vi "final_usrp_transceiver.vi"() -> ()   [LabVIEW 2014]
uses:
  <vilib>/vision/Image Controls.llb/IMAQ Image.ctl
  <vilib>/addons/Modulation/Analog/support/mod_Set Error Source.vi
  var_stop.vi
  <vilib>/addons/Modulation/Digital/Support/Common/Validators/mod_Generate Filter Coefficients Validate.vi
  <vilib>/addons/Modulation/Digital/General/subVIs/mod_Generate Filter Coefficients.vi
  <vilib>/measure/maspectr.llb/FFT Power Spectrum and PSD for 1 Chan (CDB).vi
  <vilib>/addons/Modulation/Digital/General/MT Apply Matched Filter (Generic).vi
  <vilib>/addons/Modulation/Digital/General/MT Align to Ideal Symbols (Generic).vi
  <instrlib>/niUSRP/niUSRP Fetch Rx Data (CDB Cluster).vi
  <instrlib>/niUSRP/niUSRP Write Tx Data (CDB Cluster).vi
  <vilib>/addons/Modulation/Digital/General/MT Apply Pulse Shaping Filter (Generic).vi
  <vilib>/addons/Modulation/niDMT.lvlib
  <vilib>/measure/NI_MAPro.lvlib
panel:
  out "size(s) 4":i32
  out "length 2":i32
  out "frame num":u32
  out "length":i32[](array[numeric])
  out "start index":i32[](array[numeric])
  out "Numeric":i32
  out "size(s) 3":i32
  out "# elements in queue 2":i32
  out "size(s) 2":i32
  out "size(s)":i32[](array[numeric])
  out "image":T1(plugin-control)
  in  "Transmit power (db)":dbl
  out "found?":bool
  out "# elements in queue":i32
  out "Spectrum monitor":cluster{"f0":dbl, "df":dbl, "magnitude":dbl[]}(graph)={"f0"=-0.49993781867926873, "df"=0.00012436264146250465, "magnitude"=[]}
  out "RX Constellation Map":cdb[](graph)
  out "valid?":bool
  in  "Gray code?":bool
  in  "Modulation":enum16{"PSK", "QAM"}(ring)=enum."QAM"
  out "packet len":u32
  in  "filter length (symbols)":i32=8
  in  "filter parameter":dbl=0.5 format="%.2f"
  in  "pulse shaping filter (none)":T2(ring)=enum."Raised Cosine"
  in  "M-PSK (4)":i32=16 caption="M-ARY"
  in  "samples per symbol (16)":i32=4
  out "packet bits length":i32
  in  "number of samples":i64=40000
  out "RX coerced gain":dbl format="%#_6f"
  out "RX coerced carrier frequency":dbl=915000000.0 format="%#_6p"
  out "RX coerced IQ rate":dbl=4000000.0 format="%#_6p"
  in  "RX active antenna":string="RX2"
  in  "RX gain":dbl format="%#_6f"
  in  "RX device names":refnum<k15>="192.168.10.2"
  out "TX coerced gain":dbl format="%#_6f"
  out "TX coerced carrier frequency":dbl=915000000.0 format="%#_6p"
  out "coerced IQ rate":dbl=4000000.0 format="%#_6p"
  in  "TX device names":refnum<k15>="192.168.10.2"
  in  "TX gain":dbl format="%#_6f"
  in  "carrier frequency":dbl=915000000.0 format="%#_6p"
  in  "IQ rate":dbl=800000.0 format="%#_6p"
  in  "stop":bool
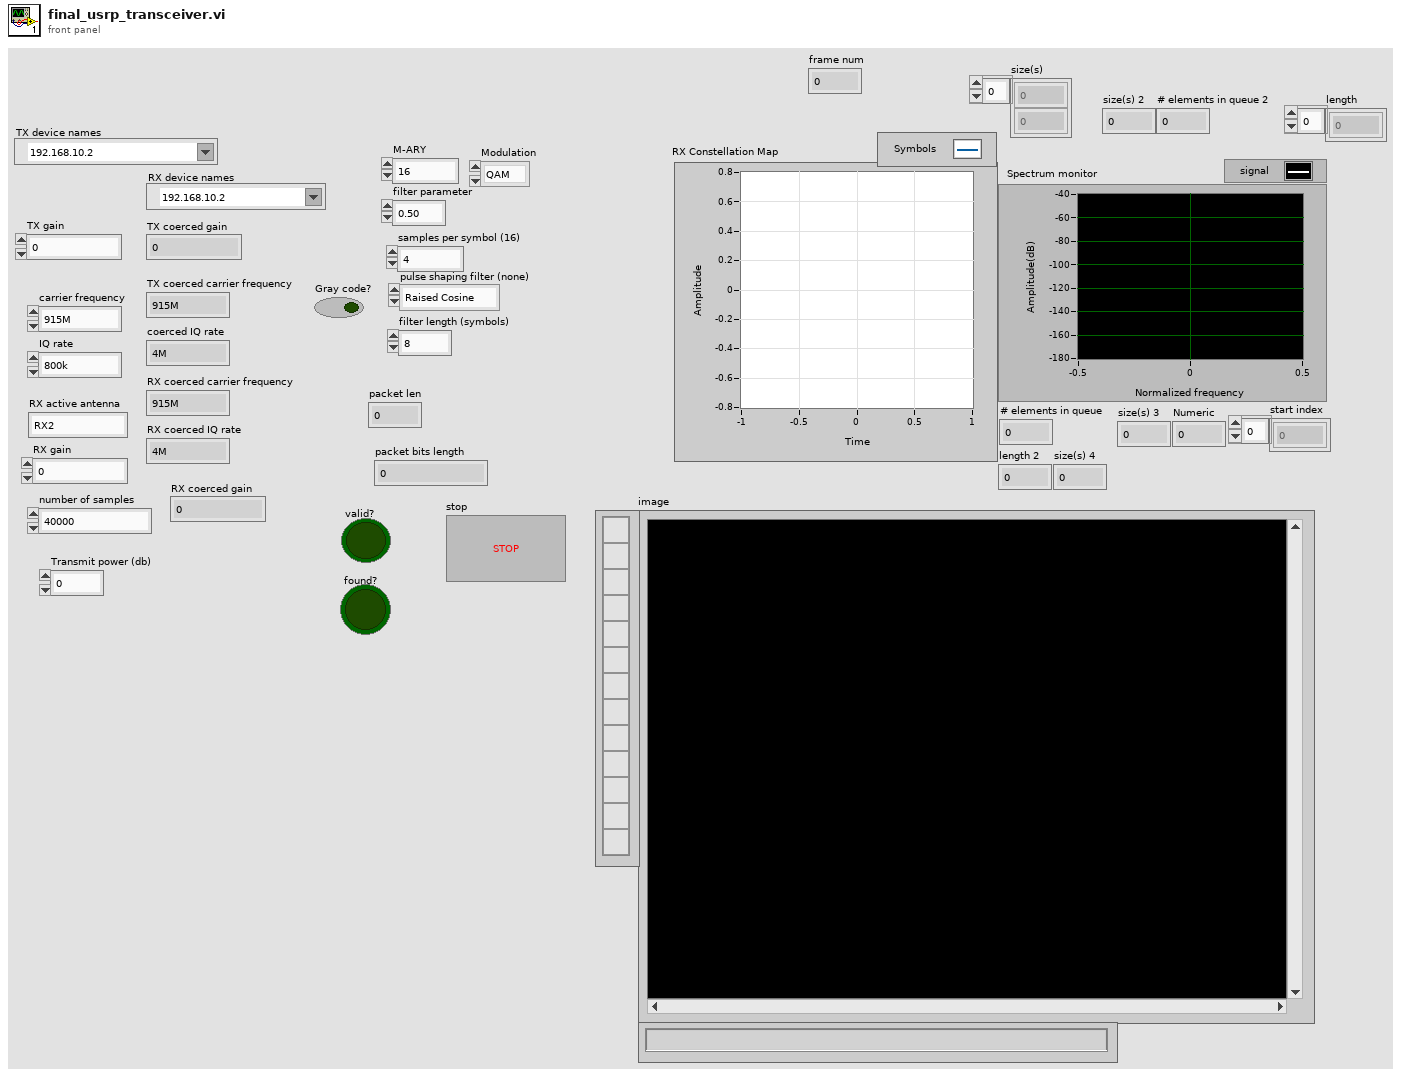
[diagram p1: front panel]
types:
  T1 = typedef "IMAQ Image.ctl" = refnum<image>
  T2 = enum16{"none", "Raised Cosine", "Root Raised Cos", "Gaussian"}
  T3 = enum16{"FSK", "PSK", "QAM", "MSK", "PAM", "ASK", "CPM"}
  T4 = cluster{"samples per symbol (16)":i32, "symbol map":cdb[], "index map":u32[]}
  T5 = cluster{"samples per symbol (16)":i32, "symbol map":cdb[], i32[]}
  T6 = typedef "niAMT.lvlib/Complex Data Waveform.ctl" = cluster{"t0":dbl, "dt":dbl, "Y":cdb[]}
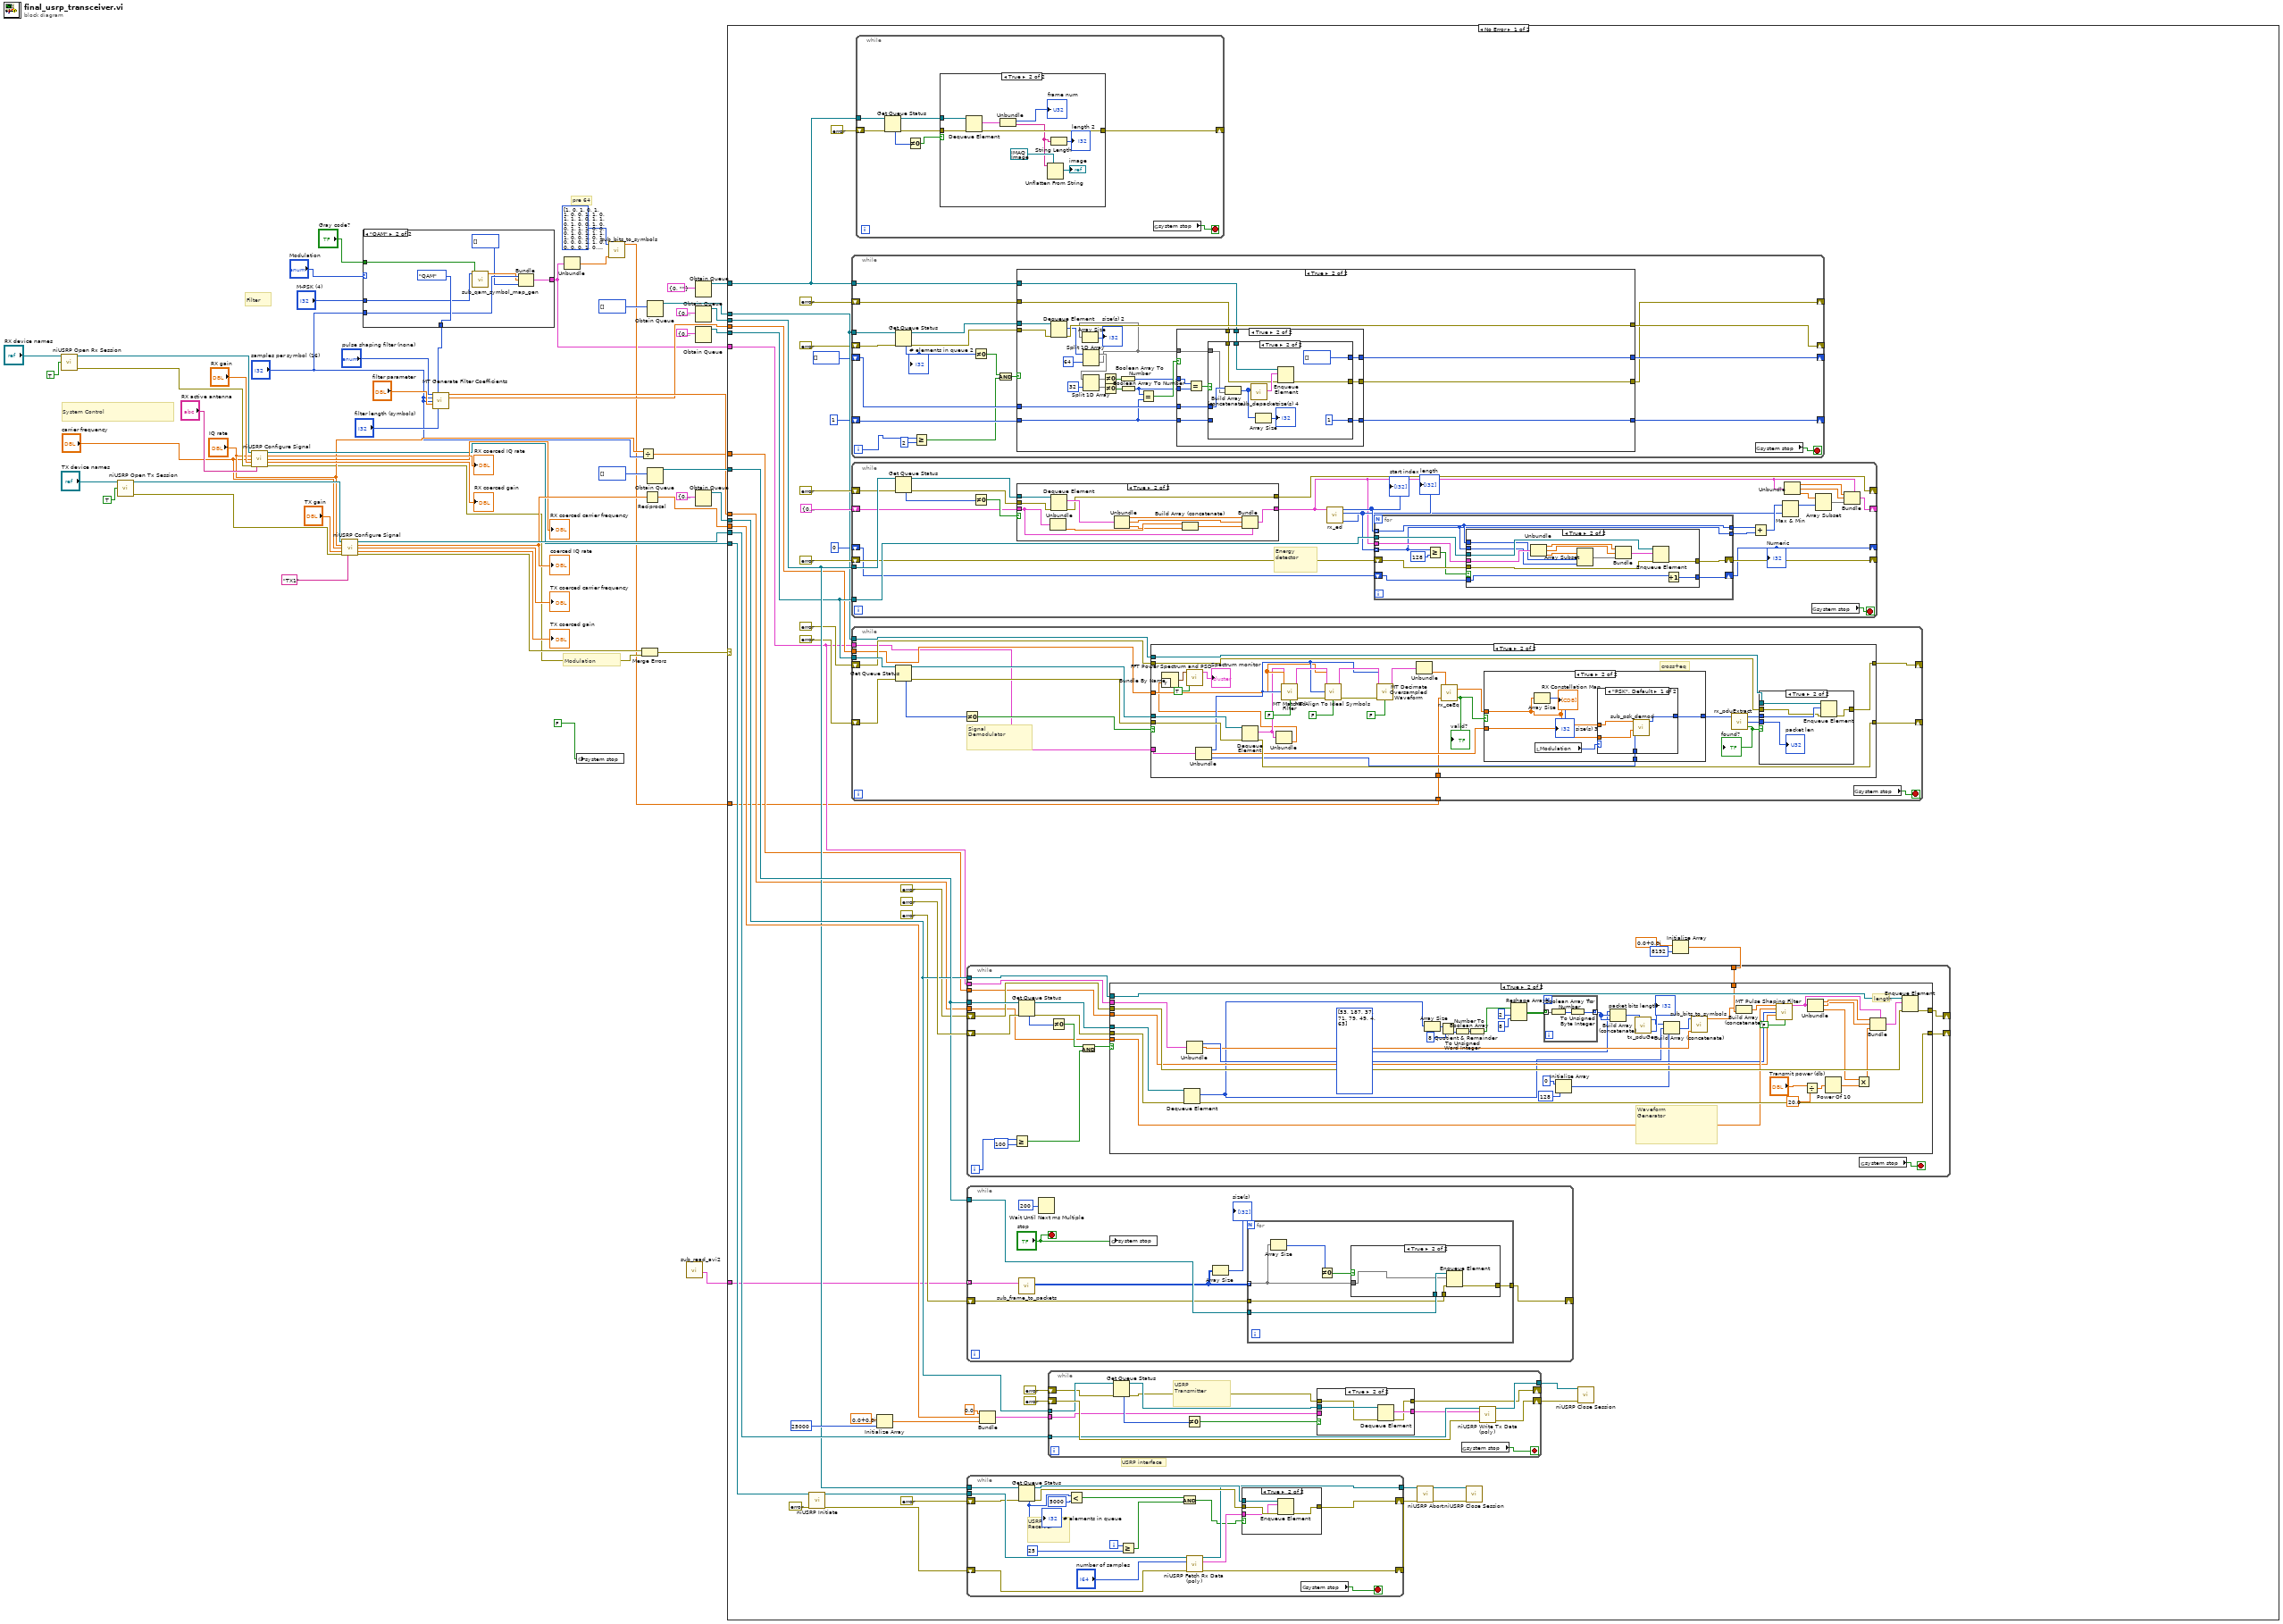
[diagram p0: block diagram]
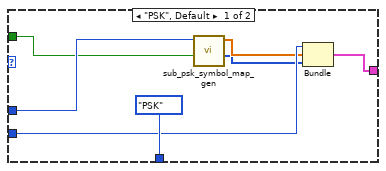
[diagram p2: hidden frame]
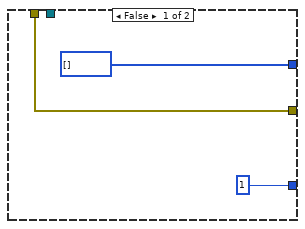
[diagram p5: hidden frame]
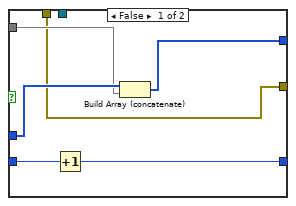
[diagram p6: hidden frame]
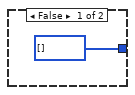
[diagram p8: hidden frame]
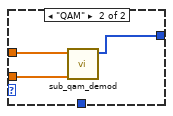
[diagram p9: hidden frame]
diagram:
  # "pre 64"
  # "Modulation"
  # "Filter"
  # "System Control"
  n1 = call <instrlib>:"niUSRP Open Rx Session.vi"("device names"="RX device names", "reset"=TRUE) -> ("session handle out"=w41:refnum<k15>, "error out"=w40:errorcluster)  [unwired: 12 in]
  n2 = call <instrlib>:"niUSRP Open Tx Session.vi"("device names"="TX device names", "reset"=TRUE) -> ("session handle out"=w54:refnum<k15>, "error out"=w53:errorcluster)  [unwired: 12 in]
  n3 = call <instrlib>:"niUSRP Configure Signal.vi"("session handle"=w41, "IQ rate"="IQ rate", "carrier frequency"="carrier frequency", "gain"="RX gain", "error in (no error)"=w40, "active antenna"="RX active antenna") -> ("session handle out"=w32:refnum<k15>, "coerced IQ rate"=→"RX coerced IQ rate":dbl, "coerced carrier frequency"=→"RX coerced carrier frequency":dbl, "coerced gain"=→"RX coerced gain":dbl, "error out"=w16:errorcluster)  [unwired: 5 in]
  n4 = call <instrlib>:"niUSRP Configure Signal.vi"("session handle"=w54, "IQ rate"="IQ rate", "carrier frequency"="carrier frequency", "gain"="TX gain", "error in (no error)"=w53, "active antenna"="TX1") -> ("session handle out"=w45:refnum<k15>, "coerced IQ rate"=w43:dbl, "coerced carrier frequency"=→"TX coerced carrier frequency":dbl, "coerced gain"=→"TX coerced gain":dbl, "error out"=w17:errorcluster)  [unwired: 5 in]
  "coerced IQ rate" <- w43
  n5 = case shown="\"QAM\"" "Modulation" {
    tunnel: [T3."PSK" ("modulation type") T3."QAM" ("modulation type")] -> w11
    tunnel: "M-PSK (4)" -> [w61 w67]
    tunnel: "Gray code?" -> [w60 w68]
    tunnel: "samples per symbol (16)" -> [w59 w66]
    tunnel: [w56 w63] -> w4
    frame "PSK", Default {
      n6 = call "sub_psk_symbol_map_gen.vi"("Gray code?"=w60, "M-PSK"=w61) -> ("index map"=w57:u32[], "symbol map"=w58:cdb[])  [unwired: 8 in]
      n7 = Bundle("samples per symbol (16)"=w59, "symbol map"=w58, "index map"=w57) -> (w56:T4)  [unwired: 1 in]
    }
    frame "QAM" {
      n8 = call "sub_qam_symbol_map_gen.vi"("Gray code?"=w68, "M-QAM"=w67) -> ("symbol map"=w65:cdb[])  [unwired: 9 in]
      n9 = Bundle("samples per symbol (16)"=w66, "symbol map"=w65, i32[] []) -> (w63:T5)  [unwired: 1 in]
    }
  }
  n10 = call <vilib>:"MT Generate Filter Coefficients.vi"("pulse shaping filter (none)"="pulse shaping filter (none)", "modulation type"=w11, "pulse shaping samples per symbol (16)"="samples per symbol (16)", "matched samples per symbol (16)"="samples per symbol (16)", "filter parameter"="filter parameter", "filter length (symbols)"="filter length (symbols)") -> ("pulse shaping filter coefficients"=w22:dbl[], "matched filter coefficients"=w20:dbl[])  [unwired: 7 in, 1 out]
  n11 = Unbundle(w4) -> ("symbol map"=w6:cdb[])  [unwired: 2 out]
  n12 = global write "var_stop.vi" "system stop"(FALSE) -> ()
  n13 = call "sub_bits_to_symbols.vi"("symbol map"=w6, "bits"=i16[] [1, 0, 1, 0, 1, 1, 0, 0, 1, 1, 0, 1, 1, 1, 0, 1, 1, 0, 1, 0, 0, 1, 0, 0, 1, 1, 1, 0, 0, 0, 1, 0, 1, 1, 1, 1, 0, 0, 1, 0, 1, 0, 0, 0, 1, 1, 0, 0, 0, 0, 1, 0, 0, 0, 0, 0, 1, 1, 1, 1, 1, 1, 0, 0] ("preamble(64) 2")) -> ("symbols"=w5:cdb[])  [unwired: 9 in]
  n14 = Divide(x="IQ rate", y="samples per symbol (16)") -> (x/y=w21:dbl)
  n15 = Merge Errors(w17, w16) -> (w15:errorcluster)
  n16 = Reciprocal(x=w43) -> (1/x=w42:dbl)
  n17 = Obtain Queue(element data type=i8[] [] ("output bit stream")) -> (queue out=w27:refnum<queue>)  [unwired: 4 in, 2 out]
  n18 = Obtain Queue(element data type=i16[] []) -> (queue out=w55:refnum<queue>)  [unwired: 4 in, 2 out]
  n19 = call "sub_read_avi2.vi"() -> ("frames"=w3:cluster{i32, "Data String":string}[])  [unwired: 10 in, 1 out]
  n20 = Obtain Queue(element data type=cluster{u32, "string":string} {0, "string"=""} ("frame")) -> (queue out=w1:refnum<queue>)  [unwired: 4 in, 2 out]
  n21 = Obtain Queue(element data type=cluster{"t0":dbl, "dt":dbl, "Y":cdb[]} {"t0"=0.0, "dt"=0.0, "Y"=[]} ("data")) -> (queue out=w31:refnum<queue>)  [unwired: 4 in, 2 out]
  n22 = Obtain Queue(element data type=cluster{"t0":dbl, "dt":dbl, "Y":cdb[]} {"t0"=0.0, "dt"=0.0, "Y"=[]} ("data")) -> (queue out=w28:refnum<queue>)  [unwired: 4 in, 2 out]
  n23 = Obtain Queue(element data type=cluster{"t0":dbl, "dt":dbl, "Y":cdb[]} {"t0"=0.0, "dt"=1.0, "Y"=[]} ("data")) -> (queue out=w46:refnum<queue>)  [unwired: 4 in, 2 out]
  n24 = case shown="No Error" w15 {
    tunnel: w55 -> [w117 _]
    tunnel: w46 -> [w112 _]
    tunnel: w45 -> [w113 _]
    tunnel: w42 -> [w106 _]
    tunnel: w32 -> [w101 _]
    tunnel: w31 -> [w95 _]
    tunnel: w28 -> [w91 _]
    tunnel: w27 -> [w89 _]
    tunnel: w4 -> [w83 _]
    tunnel: w22 -> [w86 _]
    tunnel: w21 -> [w85 _]
    tunnel: w20 -> [w84 _]
    tunnel: w5 -> [w77 _]
    tunnel: w3 -> [w76 _]
    tunnel: w1 -> [w72 _]
    frame No Error {
      # "USRP interface"
      n25 = call <instrlib>:"niUSRP Initiate.vi"("session handle"=w101, "error in (no error)"=errorcluster {"status"=FALSE, "code"=0, "source"=""}) -> ("session handle out"=w100:refnum<k15>, "error out"=w99:errorcluster)  [unwired: 12 in]
      n26 = while {
        tunnel: w89 -> [w155]
        shift-right: [w148] -> _
        shift-left: errorcluster {"status"=FALSE, "code"=0, "source"=""} ("error out") -> [w154]
        shift-right: [w146] -> _
        shift-left: u32 1 -> [w147]
        shift-right: [w145] -> _
        shift-left: i8[] [] ("second subarray") -> [w144]
        tunnel: w72 -> [w143]
        shift-right: [w141] -> _
        shift-left: errorcluster {"status"=FALSE, "code"=0, "source"=""} ("error out") -> [w142]
        i -> [w139]
        stop <- w153 stop-if-true
        n27 = Get Queue Status(queue=w155, error in (no error)=w154) -> (queue out=w150:refnum<queue>, error out=w149:errorcluster, # elements in queue=w152:i32)  [unwired: 1 in, 5 out]
        "# elements in queue 2" <- w152
        n28 = Greater Or Equal?(x=w139, y=2) -> (x >= y?=w138:bool)
        n29 = Not Equal To 0?(x=w152) -> (x != 0?=w151:bool)
        n30 = And(x=w151, y=w138) -> (x .and. y?=w137:bool)
        n31 = case shown="True" w137 {
          tunnel: w150 -> [_ w182]
          tunnel: w149 -> [w159 w181]
          tunnel: [w159 w180] -> w148
          tunnel: w147 -> [w158 w166]
          tunnel: [w158 w167] -> w146
          tunnel: [w156 w171] -> w145
          tunnel: w144 -> [w156 w168]
          tunnel: w143 -> [_ w165]
          tunnel: w142 -> [w157 w164]
          tunnel: [w157 w163] -> w141
          frame False {
          }
          frame True {
            n32 = Dequeue Element(queue=w182, error in (no error)=w181) -> (element=w162:i8[], error out=w180:errorcluster)  [unwired: 1 in, 2 out]
            n33 = Split 1D Array(array=w162, index=64) -> (first subarray=w173:i8[], second subarray=w160:i8[])
            n34 = Array Size(array=w160) -> (size(s)=→"size(s) 2":i32)
            n35 = Split 1D Array(array=w173, index=32) -> (first subarray=w176:i8[], second subarray=w177:i8[])
            n36 = Not Equal To 0?(x=w176) -> (x != 0?=w175:bool[])
            n37 = Not Equal To 0?(x=w177) -> (x != 0?=w174:bool[])
            n38 = Boolean Array To Number(Boolean array=w175) -> (number=w170:u32)
            n39 = Boolean Array To Number(Boolean array=w174) -> (number=w169:u32)
            n40 = Equal?(x=w169, y=w166) -> (x = y?=w172:bool)
            n41 = case shown="True" w172 {
              tunnel: [i8[] [] ("second subarray") w193] -> w171
              tunnel: w170 -> [_ w196]
              tunnel: w169 -> [_ w195]
              tunnel: w168 -> [_ w192]
              tunnel: w160 -> [_ w191]
              tunnel: [u32 1 w190] -> w167
              tunnel: w166 -> [_ w189]
              tunnel: w165 -> [_ w188]
              tunnel: w164 -> [w183 w187]
              tunnel: [w183 w186] -> w163
              frame False {
              }
              frame True {
                n42 = Equal?(x=w196, y=w195) -> (x = y?=w194:bool)
                n43 = case shown="True" w194 {
                  tunnel: [w200 i8[] [] ("second subarray")] -> w193
                  tunnel: w192 -> [w202 w210]
                  tunnel: w191 -> [w201 w209]
                  tunnel: [w198 u32 1] -> w190
                  tunnel: w189 -> [w199 _]
                  tunnel: w188 -> [_ w208]
                  tunnel: w187 -> [w197 w206]
                  tunnel: [w197 w205] -> w186
                  frame False {
                    n44 = Increment(x=w199) -> (x+1=w198:u32)
                    n45 = Build Array (concatenate)(w202, w201) -> (w200:i8[])
                  }
                  frame True {
                    n46 = Build Array (concatenate)(w210, w209) -> (w204:i8[])
                    n47 = call "sub_depacket.vi"("bitstream"=w204) -> ("frame"=w207:cluster{u32, "string":string})  [unwired: 10 in]
                    n48 = Array Size(array=w204) -> (size(s)=→"size(s) 4":i32)
                    n49 = Enqueue Element(queue=w208, element=w207, error in (no error)=w206) -> (error out=w205:errorcluster)  [unwired: 1 in, 2 out]
                  }
                }
              }
            }
          }
        }
        n50 = global read "var_stop.vi" "system stop"() -> (w153:bool)
      }
      n51 = while {
        tunnel: w95 -> [w307]
        shift-right: [w300] -> _
        shift-left: errorcluster {"status"=FALSE, "code"=0, "source"=""} ("error out") -> [w306]
        shift-right: [w286] -> _
        shift-left: cluster{"t0":dbl, "dt":dbl, "Y":cdb[]} {"t0"=0.0, "dt"=0.0, "Y"=[]} ("data") -> [w301]
        tunnel: w91 -> [w299]
        shift-right: [w298] -> _
        shift-left: errorcluster {"status"=FALSE, "code"=0, "source"=""} ("error out") -> [w297]
        shift-right: [w281] -> _
        shift-left: 0 -> [w282]
        stop <- w296 stop-if-true
        # "Energy\ndetector"
        n52 = Get Queue Status(queue=w307, error in (no error)=w306) -> (queue out=w302:refnum<queue>, error out=w303:errorcluster, # elements in queue=w305:i32)  [unwired: 1 in, 5 out]
        n53 = Not Equal To 0?(x=w305) -> (x != 0?=w304:bool)
        n54 = case shown="True" w304 {
          tunnel: w303 -> [w334 w345]
          tunnel: w302 -> [_ w344]
          tunnel: w301 -> [w333 w339]
          tunnel: [w334 w336] -> w300
          tunnel: [w333 w335] -> w293
          frame False {
          }
          frame True {
            n55 = Unbundle(w339) -> ("Y"=w342:cdb[])  [unwired: 2 out]
            n56 = Dequeue Element(queue=w344, error in (no error)=w345) -> (element=w343:cluster{"t0":dbl, "dt":dbl, "Y":cdb[]}, error out=w336:errorcluster)  [unwired: 1 in, 2 out]
            n57 = Unbundle(w343) -> ("t0"=w338:dbl, "dt"=w337:dbl, "Y"=w341:cdb[])
            n58 = Build Array (concatenate)(w342, w341) -> (w340:cdb[])
            n59 = Bundle(cluster=w339, "t0"=w338, "dt"=w337, "Y"=w340) -> (w335:cluster{"t0":dbl, "dt":dbl, "Y":cdb[]})
          }
        }
        n60 = call "rx_ed.vi"("Wavefrom"=w293) -> ("first pulse"=w283:i32, "length"=w294:i32[], "start index"=w295:i32[])  [unwired: 8 in]
        "start index" <- w295
        "length" <- w294
        n61 = for {
          tunnel: w299 -> [w317]
          tunnel: w293 -> [w314]
          shift-right: [w316] -> w298
          shift-left: w297 -> [w315]
          tunnel: w295 -> [w313] mode=indexing
          tunnel: w294 -> [w312] mode=indexing
          tunnel: [w313] -> w289
          tunnel: [w312] -> w288
          shift-right: [w308] -> w281
          shift-left: w282 -> [w309]
          n62 = Greater Or Equal?(x=w312, y=128) -> (x >= y?=w310:bool)
          n63 = case shown="True" w310 {
            tunnel: w317 -> [_ w332]
            tunnel: [w319 w331] -> w316
            tunnel: w315 -> [w319 w330]
            tunnel: w314 -> [_ w329]
            tunnel: w313 -> [_ w323]
            tunnel: w312 -> [_ w322]
            tunnel: w309 -> [w318 w321]
            tunnel: [w318 w320] -> w308
            frame False {
            }
            frame True {
              n64 = Unbundle(w329) -> ("t0"=w327:dbl, "dt"=w328:dbl, "Y"=w325:cdb[])
              n65 = Array Subset(array=w325, index=w323, length=w322) -> (w324:cdb[])
              n66 = Bundle("t0"=w327, "dt"=w328, w324) -> (w326:cluster{"t0":dbl, "dt":dbl, cdb[]})  [unwired: 1 in]
              n67 = Enqueue Element(queue=w332, element=w326, error in (no error)=w330) -> (error out=w331:errorcluster)  [unwired: 1 in, 2 out]
              n68 = Increment(x=w321) -> (x+1=w320:i32)
            }
          }
        }
        "Numeric" <- w281
        n69 = Add(x=w289, y=w288) -> (x+y=w285:i32)
        n70 = Max & Min(x=w285, y=w283) -> (max(x,y)=w284:i32)  [unwired: 1 out]
        n71 = Unbundle(w293) -> ("t0"=w292:dbl, "dt"=w291:dbl, "Y"=w290:cdb[])
        n72 = global read "var_stop.vi" "system stop"() -> (w296:bool)
        n73 = Array Subset(array=w290, index=w284) -> (w287:cdb[])  [unwired: 1 in]
        n74 = Bundle(cluster=w293, "t0"=w292, "dt"=w291, "Y"=w287) -> (w286:cluster{"t0":dbl, "dt":dbl, "Y":cdb[]})
      }
      n75 = while {
        tunnel: w91 -> [w226]
        shift-right: [w220] -> _
        shift-left: errorcluster {"status"=FALSE, "code"=0, "source"=""} ("error out") -> [w225]
        tunnel: w89 -> [w219]
        shift-right: [w218] -> _
        shift-left: errorcluster {"status"=FALSE, "code"=0, "source"=""} ("error out") -> [w217]
        tunnel: w84 -> [w215]
        tunnel: w83 -> [w214]
        tunnel: w77 -> [w213]
        stop <- w216 stop-if-true
        # "Signal \nDemodulator"
        n76 = Get Queue Status(queue=w226, error in (no error)=w225) -> (queue out=w222:refnum<queue>, error out=w221:errorcluster, # elements in queue=w224:i32)  [unwired: 1 in, 5 out]
        n77 = Not Equal To 0?(x=w224) -> (x != 0?=w223:bool)
        n78 = case shown="True" w223 {
          tunnel: w222 -> [_ w259]
          tunnel: w221 -> [w228 w260]
          tunnel: [w228 w258] -> w220
          tunnel: w219 -> [_ w248]
          tunnel: [w227 w247] -> w218
          tunnel: w217 -> [w227 w246]
          tunnel: w215 -> [_ w235]
          tunnel: w214 -> [_ w239]
          tunnel: w213 -> [_ w231]
          frame False {
          }
          frame True {
            # "cross+eq"
            n79 = Unbundle(w239) -> ("samples per symbol (16)"=w238:i32, "symbol map"=w237:cdb[], "index map"=w236:u32[])
            n80 = Dequeue Element(queue=w259, error in (no error)=w260) -> (element=w230:cluster{"t0":dbl, "dt":dbl, "Y":cdb[]}, error out=w258:errorcluster)  [unwired: 1 in, 2 out]
            n81 = Unbundle(w230) -> ("Y"=w229:cdb[])  [unwired: 2 out]
            n82 = Bundle By Name("Y"=w229) -> (w234:waveform(cdb))  [unwired: 1 in]
            n83 = call-poly <vilib>:"FFT Power Spectrum and PSD.vi"("dB On (F)"=TRUE, "time signal"=w234) -> ("Power Spectrum / PSD"=→"Spectrum monitor":cluster{"f0":dbl, "df":dbl, "magnitude":dbl[]})  [unwired: 6 in, 3 out]
            n84 = call-poly <vilib>:"MT Matched Filter.vi"("input complex waveform"=w230, "matched filter coefficients"=w235, "samples per symbol (16)"=w238, "reset? (T)"=FALSE) -> ("output complex waveform"=w257:T6, "error out"=w256:errorcluster)  [unwired: 10 in]
            n85 = call-poly <vilib>:"MT Align To Ideal Symbols.vi"("input complex waveform"=w257, "matched filter coefficients"=w235, "samples per symbol (16)"=w238, "error in (no error)"=w256, "reset? (T)"=FALSE) -> ("output complex waveform"=w254:T6, "error out"=w255:errorcluster)  [unwired: 8 in, 1 out]
            n86 = call <vilib>:"MT Decimate Oversampled Waveform.vi"("input complex waveform"=w254, "decimation factor"=w238, "error in (no error)"=w255, "reset? (T)"=FALSE) -> ("output complex waveform"=w253:T6)  [unwired: 10 in, 1 out]
            n87 = Unbundle(w253) -> ("Y"=w249:cdb[])  [unwired: 2 out]
            n88 = call "rx_ceEq.vi"("preamble"=w231, "symbols"=w249) -> ("valid?"=w244:bool, "eq symbols"=w245:cdb[])
            "valid?" <- w244
            n89 = case shown="True" w244 {
              tunnel: [i8[] [] ("output bit stream") w265] -> w252
              tunnel: w237 -> [_ w266]
              tunnel: w245 -> [_ w263]
              tunnel: w236 -> [_ w264]
              frame False {
              }
              frame True {
                n90 = Array Size(array=w263) -> (size(s)=→"size(s) 3":i32)
                n91 = local read "Modulation"() -> (w267:enum16{"PSK", "QAM"})
                n92 = case shown="\"PSK\", Default" w267 {
                  tunnel: w263 -> [w271 w274]
                  tunnel: w266 -> [w270 w273]
                  tunnel: [w268 w272] -> w265
                  tunnel: w264 -> [w269 _]
                  frame "PSK", Default {
                    n93 = call "sub_psk_demod.vi"("index map"=w269, "symbol map"=w270, "symbol"=w271) -> ("bitstream"=w268:i16[])  [unwired: 8 in]
                  }
                  frame "QAM" {
                    n94 = call "sub_qam_demod.vi"("symbol map"=w273, "symbol"=w274) -> ("bitstream"=w272:i16[])  [unwired: 9 in]
                  }
                }
                "RX Constellation Map" <- w263
              }
            }
            n95 = call "rx_pduExtract.vi"("output bit stream"=w252) -> ("found?"=w251:bool, "packet len"=w243:u32, "ppdu"=w250:i8[])  [unwired: 2 in]
            "found?" <- w251
            n96 = case shown="True" w251 {
              tunnel: w250 -> [_ w278]
              tunnel: w248 -> [_ w280]
              tunnel: [w275 w279] -> w247
              tunnel: w246 -> [w275 w276]
              tunnel: w243 -> [_ w277]
              frame False {
              }
              frame True {
                n97 = Enqueue Element(queue=w280, element=w278, error in (no error)=w276) -> (error out=w279:errorcluster)  [unwired: 1 in, 2 out]
                "packet len" <- w277
              }
            }
          }
        }
        n98 = global read "var_stop.vi" "system stop"() -> (w216:bool)
      }
      n99 = while {
        tunnel: w72 -> [w126]
        shift-right: [w120] -> _
        shift-left: errorcluster {"status"=FALSE, "code"=0, "source"=""} ("error out") -> [w125]
        stop <- w119 stop-if-true
        n100 = Get Queue Status(queue=w126, error in (no error)=w125) -> (queue out=w122:refnum<queue>, error out=w121:errorcluster, # elements in queue=w124:i32)  [unwired: 1 in, 5 out]
        n101 = Not Equal To 0?(x=w124) -> (x != 0?=w123:bool)
        n102 = case shown="True" w123 {
          tunnel: w122 -> [_ w136]
          tunnel: w121 -> [w127 w135]
          tunnel: [w127 w133] -> w120
          frame False {
          }
          frame True {
            n103 = Dequeue Element(queue=w136, error in (no error)=w135) -> (element=w134:cluster{u32, "string":string}, error out=w133:errorcluster)  [unwired: 1 in, 2 out]
            n104 = Unbundle(w134) -> (→"frame num":u32, "string"=w129:string)
            n105 = Unflatten From String(type=T1 refnum ("Image Out"), binary string=w129) -> (value=→"image":T1)  [unwired: 3 in, 2 out]
            n106 = String Length(string=w129) -> (length=→"length 2":i32)
          }
        }
        n107 = global read "var_stop.vi" "system stop"() -> (w119:bool)
      }
      n108 = Initialize Array(cdb 0.0+0.0i, 25000 ("dimension size")) -> (w107:cdb[])
      n109 = while {
        tunnel: w117 -> [w463]
        shift-right: [w461] -> _
        shift-left: errorcluster {"status"=FALSE, "code"=0, "source"=""} ("error out") -> [w462]
        tunnel: w76 -> [w460] mode=indexing
        stop <- "stop" stop-if-true
        n110 = call "sub_frame_to_packets.vi"("Cluster"=w460) -> ("packets"=w459:i16[][])  [unwired: 10 in]
        n111 = Wait Until Next ms Multiple(millisecond multiple=u32 200) -> ()  [unwired: 1 out]
        n112 = global write "var_stop.vi" "system stop"("stop") -> ()
        n113 = Array Size(array=w459) -> (size(s)=→"size(s)":i32[])
        n114 = for {
          tunnel: w463 -> [w470]
          tunnel: w462 -> [w469]
          tunnel: [w468] -> w461
          tunnel: w459 -> [w465] mode=indexing
          n115 = Array Size(array=w465) -> (size(s)=w466:i32)
          n116 = Not Equal To 0?(x=w466) -> (x != 0?=w467:bool)
          n117 = case shown="True" w467 {
            tunnel: w465 -> [_ w472]
            tunnel: w470 -> [_ w475]
            tunnel: w469 -> [w471 w474]
            tunnel: [w471 w473] -> w468
            frame False {
            }
            frame True {
              n118 = Enqueue Element(queue=w475, element=w472, error in (no error)=w474) -> (error out=w473:errorcluster)  [unwired: 1 in, 2 out]
            }
          }
        }
      }
      n119 = while {
        tunnel: w100 -> [w364]
        shift-right: [w353] -> w96
        shift-left: w99 -> [w363]
        tunnel: w95 -> [w361]
        shift-right: [w355] -> _
        shift-left: errorcluster {"status"=FALSE, "code"=0, "source"=""} ("error out") -> [w360]
        tunnel: [w354] -> w97
        i -> [w351]
        stop <- w352 stop-if-true
        # "USRP\nReceiver"
        n120 = Get Queue Status(queue=w361, error in (no error)=w360) -> (queue out=w357:refnum<queue>, error out=w356:errorcluster, # elements in queue=w359:i32)  [unwired: 1 in, 5 out]
        "# elements in queue" <- w359
        n121 = Less?(x=w359, y=5000) -> (x < y?=w349:bool)
        n122 = Greater Or Equal?(x=w351, y=25) -> (x >= y?=w348:bool)
        n123 = And(x=w349, y=w348) -> (x .and. y?=w346:bool)
        n124 = call-poly <instrlib>:"niUSRP Fetch Rx Data (poly).vi"("session handle"=w364, "number of samples"="number of samples", "error in (no error)"=w363) -> ("session handle out"=w354:refnum<k15>, "data"=w347:cluster{"t0":dbl, "dt":dbl, "Y":cdb[]}, "error out"=w353:errorcluster)  [unwired: 9 in, 1 out]
        n125 = case shown="True" w346 {
          tunnel: w357 -> [_ w369]
          tunnel: w356 -> [w365 w368]
          tunnel: [w365 w367] -> w355
          tunnel: w347 -> [_ w366]
          frame False {
          }
          frame True {
            n126 = Enqueue Element(queue=w369, element=w366, error in (no error)=w368) -> (error out=w367:errorcluster)  [unwired: 1 in, 2 out]
          }
        }
        n127 = global read "var_stop.vi" "system stop"() -> (w352:bool)
      }
      n128 = Bundle(0.0, w106, w107) -> (w104:cluster{dbl, dbl, cdb[]})  [unwired: 1 in]
      n129 = while {
        shift-right: [w379] -> w116
        shift-left: errorcluster {"status"=FALSE, "code"=0, "source"=""} ("error out") -> [w377]
        tunnel: [w378] -> w115
        tunnel: w113 -> [w376]
        tunnel: w112 -> [w374]
        shift-right: [w372] -> _
        shift-left: errorcluster {"status"=FALSE, "code"=0, "source"=""} ("error out") -> [w373]
        tunnel: w104 -> [w371]
        stop <- w370 stop-if-true
        # "USRP\nTransmitter"
        n130 = Get Queue Status(queue=w374, error in (no error)=w373) -> (queue out=w381:refnum<queue>, error out=w380:errorcluster, # elements in queue=w383:i32)  [unwired: 1 in, 5 out]
        n131 = Not Equal To 0?(x=w383) -> (x != 0?=w382:bool)
        n132 = case shown="True" w382 {
          tunnel: w381 -> [_ w389]
          tunnel: w380 -> [w384 w388]
          tunnel: [w385 w387] -> w375
          tunnel: [w384 w386] -> w372
          tunnel: w371 -> [w385 _]
          frame False {
          }
          frame True {
            n133 = Dequeue Element(queue=w389, error in (no error)=w388) -> (element=w387:cluster{"t0":dbl, "dt":dbl, "Y":cdb[]}, error out=w386:errorcluster)  [unwired: 1 in, 2 out]
          }
        }
        n134 = global read "var_stop.vi" "system stop"() -> (w370:bool)
        n135 = call-poly <instrlib>:"niUSRP Write Tx Data (poly).vi"("session handle"=w376, "data"=w375, "error in (no error)"=w377) -> ("session handle out"=w378:refnum<k15>, "error out"=w379:errorcluster)  [unwired: 11 in]
      }
      n136 = call <instrlib>:"niUSRP Abort.vi"("session handle"=w97, "error in (no error)"=w96) -> ("session handle out"=w103:refnum<k15>, "error out"=w102:errorcluster)  [unwired: 12 in]
      n137 = call <instrlib>:"niUSRP Close Session.vi"("session handle"=w103, "error in (no error)"=w102) -> ()  [unwired: 13 in, 1 out]
      n138 = call <instrlib>:"niUSRP Close Session.vi"("session handle"=w115, "error in (no error)"=w116) -> ()  [unwired: 13 in, 1 out]
      n139 = Initialize Array(cdb 0.0+0.0i, 8192 ("dimension size")) -> (w78:cdb[])
      n140 = while {
        tunnel: w117 -> [w405]
        shift-right: [w402] -> _
        shift-left: errorcluster {"status"=FALSE, "code"=0, "source"=""} ("error out") -> [w408]
        tunnel: w112 -> [w401]
        shift-right: [w400] -> _
        shift-left: errorcluster {"status"=FALSE, "code"=0, "source"=""} ("error out") -> [w399]
        tunnel: w83 -> [w397]
        tunnel: w86 -> [w396]
        tunnel: w85 -> [w395]
        tunnel: w78 -> [w394]
        i -> [w393]
        stop <- w398 stop-if-true
        n141 = Greater Or Equal?(x=w393, y=100) -> (x >= y?=w390:bool)
        n142 = Get Queue Status(queue=w405, error in (no error)=w408) -> (queue out=w403:refnum<queue>, error out=w404:errorcluster, # elements in queue=w407:i32)  [unwired: 1 in, 5 out]
        n143 = Not Equal To 0?(x=w407) -> (x != 0?=w406:bool)
        n144 = And(x=w406, y=w390) -> (x .and. y?=w391:bool)
        n145 = case shown="True" w391 {
          tunnel: w404 -> [w410 w453]
          tunnel: w403 -> [_ w452]
          tunnel: [w410 w451] -> w402
          tunnel: w401 -> [_ w446]
          tunnel: [w409 w445] -> w400
          tunnel: w399 -> [w409 w444]
          tunnel: w397 -> [_ w441]
          tunnel: w396 -> [_ w440]
          tunnel: w395 -> [_ w439]
          tunnel: w394 -> [_ w429]
          frame False {
          }
          frame True {
            # "length"
            # "Waveform \nGenerator"
            n146 = Dequeue Element(queue=w452, error in (no error)=w453) -> (element=w413:i16[], error out=w451:errorcluster)  [unwired: 1 in, 2 out]
            n147 = Unbundle(w441) -> ("samples per symbol (16)"=w435:i32, "symbol map"=w428:cdb[])  [unwired: 1 out]
            n148 = Array Size(array=w413) -> (size(s)=w437:i32)
            n149 = Quotient & Remainder(x=w437, y=8) -> (floor(x/y)=w417:i32)  [unwired: 1 out]
            n150 = To Unsigned Word Integer(number=w417) -> (unsigned 16bit integer=w436:u16)
            n151 = Number To Boolean Array(number=w436) -> (Boolean array=w450:bool[])
            n152 = Reshape Array(w450, 2 ("dimension size"), 8 ("dimension size")) -> (w447:bool[][])
            n153 = for {
              tunnel: w447 -> [w456] mode=indexing
              tunnel: [w454] -> w438 mode=indexing
              n154 = Boolean Array To Number(Boolean array=w456) -> (number=w455:u32)
              n155 = To Unsigned Byte Integer(number=w455) -> (unsigned 8bit integer=w454:u8)
            }
            n156 = Initialize Array(u8 0, 128 ("dimension size")) -> (w412:u8[])
            n157 = Build Array (concatenate)(u8[] [53, 187, 37, 71, 79, 49, 4, 63] ("Array 2"), w438, w438) -> (w443:u8[])
            n158 = call "tx_pduGen.vi"("byte array"=w443) -> ("packet bits length"=→"packet bits length":i32, "pdu"=w414:i32[])  [unwired: 3 in]
            n159 = Build Array (concatenate)(w414, w413, w412) -> (w411:i32[])
            n160 = call "sub_bits_to_symbols.vi"("symbol map"=w428, "bits"=w411) -> ("symbols"=w427:cdb[])  [unwired: 9 in]
            n161 = Build Array (concatenate)(w427, w429) -> (w425:cdb[])
            n162 = call-poly <vilib>:"MT Pulse Shaping Filter.vi"("symbols"=w425, "pulse shaping filter coefficients"=w440, "samples per symbol (16)"=w435, "symbol rate (Hz)"=w439, "reset? (T)"=FALSE) -> ("output complex waveform"=w434:T6)  [unwired: 9 in, 1 out]
            n163 = Divide(x="Transmit power (db)", y=20.0) -> (x/y=w422:dbl)
            n164 = Unbundle(w434) -> ("t0"=w433:dbl, "dt"=w432:dbl, "Y"=w420:cdb[])
            n165 = Power Of 10(x=w422) -> (10^x=w421:dbl)
            n166 = Multiply(x=w420, y=w421) -> (x*y=w419:cdb[])
            n167 = Bundle(cluster=w434, "t0"=w433, "dt"=w432, "Y"=w419) -> (w431:T6)
            n168 = Enqueue Element(queue=w446, element=w431, error in (no error)=w444) -> (error out=w445:errorcluster)  [unwired: 1 in, 2 out]
          }
        }
        n169 = global read "var_stop.vi" "system stop"() -> (w398:bool)
      }
    }
    frame Error {
    }
  }
